vi "Write KeeperPlay.vi"(8 "error in (no error)":errorcluster, 10 "KeeperPlay":T1=enum."NormalGame", 11 "Team in":refnum<class "Team.lvclass">) -> (0 "error out":errorcluster, 3 "Team out":refnum<class "Team.lvclass">)   [LabVIEW 2023, in "Team.lvclass"]
uses:
  Team.lvclass
  KeeperPlay.ctl
  Team.lvclass/Team.ctl
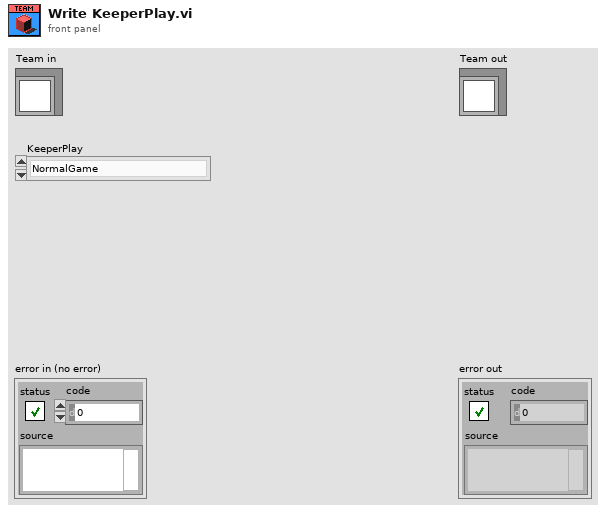
[diagram p1: front panel]
types:
  T1 = typedef "KeeperPlay.ctl" = enum16{"ZigZag", "Goto", "NormalGame", "KeeperPlay", "Halt", "Timeout", "PenaltyEnemy", "TestPlay"}
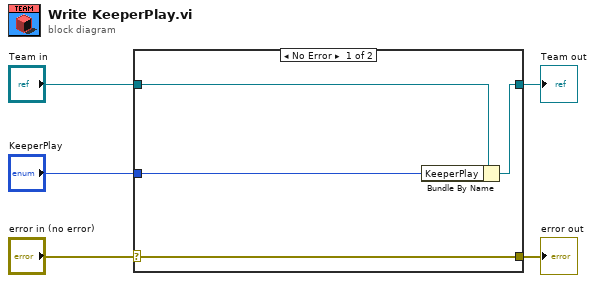
[diagram p0: block diagram]
diagram:
  n1 = case shown="No Error" "error in (no error)" {
    selector: "error in (no error)" -> [w9 w10]
    tunnel: [w9 w10] -> w4
    tunnel: [w7 w11] -> w2
    tunnel: "Team in" -> [w8 w11]
    tunnel: "KeeperPlay" -> [w6 _]
    frame No Error {
      n2 = Bundle By Name(cluster=w8, "KeeperPlay"=w6) -> (w7:refnum<class "Team.lvclass">)
    }
    frame Error {
    }
  }
  "error out" <- w4
  "Team out" <- w2
